vi "Text_New.vi"(7 "CreateMethod(Create or look up existing)":T1(ring), 8 "error in (no error)":errorcluster, 10 "Object name":string, 11 "Text In":refnum<class "Text.lvclass">) -> (0 "error out":errorcluster, 2 "DVRRefOut":refnum<data-value>, 3 "Text Out":refnum<class "Text.lvclass">, 5 "NewObjectCreated":bool)   [LabVIEW 2015, in "Front Panel Publisher.lvlib" / "Text.lvclass"]
uses:
  Text.lvclass
  Attributes.ctl
  Text.lvclass/Text.ctl
  Object_class/Object.lvclass
panel:
  in  "DVRRef(Hidden)":refnum<data-value>
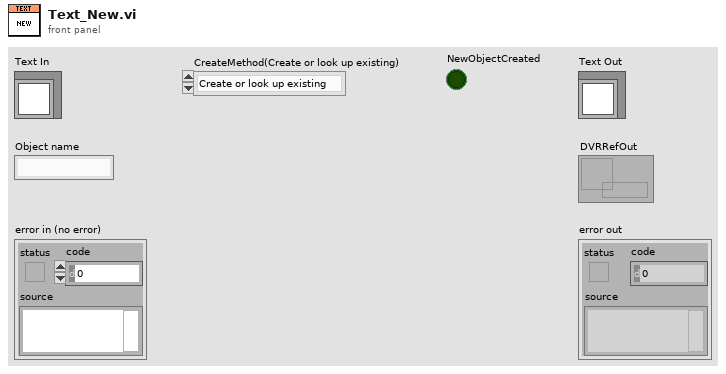
[diagram p1: front panel]
types:
  T1 = enum16{"Create or look up existing", "Look up existing"}
  T2 = typedef "Front Panel Publisher.lvlib/Text.lvclass/Attributes.ctl" = cluster{"Text":string, "Font":string, "Font Size":u32, "Visible":bool, "Control Reference":refnum<vi>}
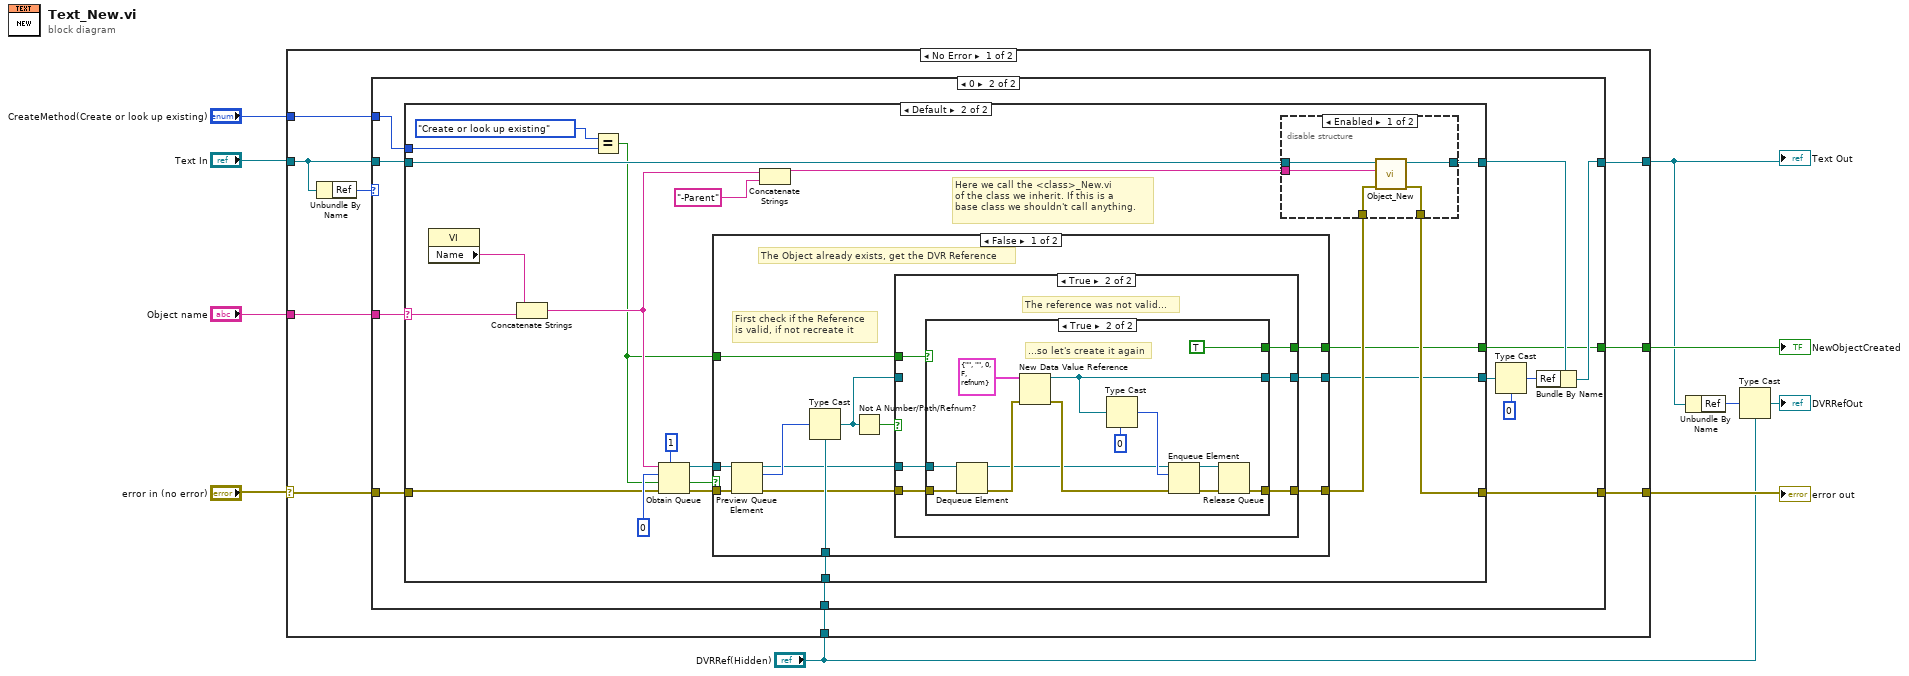
[diagram p0: block diagram]
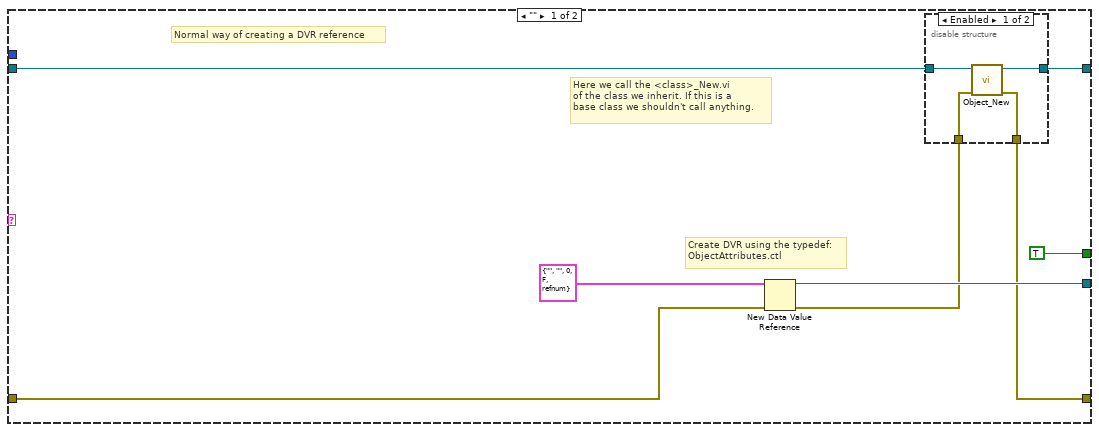
[diagram p3: hidden frame]
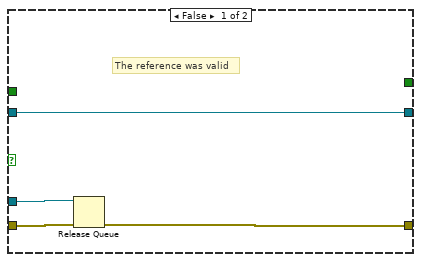
[diagram p5: hidden frame]
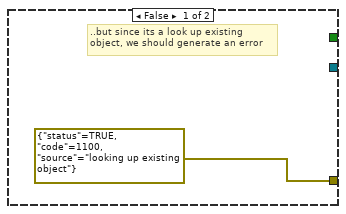
[diagram p6: hidden frame]
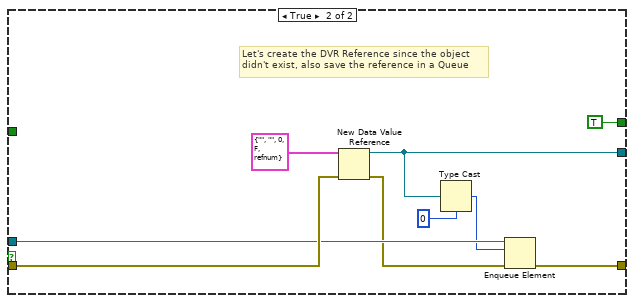
[diagram p7: hidden frame]
diagram:
  n1 = case shown="No Error" "error in (no error)" {
    selector: "error in (no error)" -> [w19 w122]
    tunnel: [w16 w122] -> w6
    tunnel: "CreateMethod(Create or look up existing)" -> [w17 _]
    tunnel: "Object name" -> [w18 _]
    tunnel: "DVRRef(Hidden)" -> [w15 _]
    tunnel: "Text In" -> [w14 w121]
    tunnel: [w13 w121] -> w3
    tunnel: [w12 _] -> w5
    frame No Error {
      n2 = Unbundle By Name(w14) -> ("Ref"=w11:u32)
      n3 = case shown="0" w11 {
        tunnel: w19 -> [w21 w33]
        tunnel: w18 -> [_ w32]
        tunnel: w17 -> [_ w31]
        tunnel: [w21 w30] -> w16
        tunnel: w14 -> [w20 w28]
        tunnel: [w20 w29] -> w13
        tunnel: w15 -> [_ w26]
        tunnel: [_ w25] -> w12
        frame Default {
          # "The DVR reference has already been created, from this child class's <Child>_New.vi"
        }
        frame 0 {
          n4 = case shown="Default" w32 {
            selector: w32 -> [_ w60]
            tunnel: w33 -> [w41 w57]
            tunnel: [w36 w58] -> w30
            tunnel: w31 -> [_ w67]
            tunnel: [w40 w51] -> w23
            tunnel: w28 -> [w39 w66]
            tunnel: [w38 w65] -> w27
            tunnel: w26 -> [_ w56]
            tunnel: [TRUE w50] -> w25
            frame "" {
              # "Create DVR using the typedef:\nObjectAttributes.ctl"
              # "Here we call the <class>_New.vi\nof the class we inherit. If this is a\nbase class we shouldn't call anything."
              # "Normal way of creating a DVR reference"
              n5 = New Data Value Reference(data value=T2 {"Text"="", "Font"="", "Font Size"=0, "Visible"=FALSE, "Control Reference"=refnum} ("Data"), error in=w41) -> (data value reference=w40:refnum<data-value>, error out=w37:errorcluster)
              n6 = disable-structure shown="Enabled" {
                disable-tunnel: w39 -> [w45 w47]
                disable-tunnel: [w44 w47] -> w38
                disable-tunnel: w37 -> [w43 w46]
                disable-tunnel: [w42 w46] -> w36
                frame Enabled {
                  n7 = call "Object_New.vi"("error in (no error)"=w43, "Object In"=w45) -> ("error out"=w42:errorcluster, "Object Out"=w44:refnum<class "Text.lvclass">)  [unwired: 6 in, 2 out]
                }
                frame Disabled {
                }
              }
            }
            frame Default {
              # "Here we call the <class>_New.vi\nof the class we inherit. If this is a\nbase class we shouldn't call anything."
              n8 = property class="VI"() -> ("Name"=w61:string)  [unwired: 2 in, 2 out]
              n9 = Concatenate Strings(w61, w60) -> (w59:string)
              n10 = Equal?(x=T1."Create or look up existing", y=w67) -> (x = y?=w49:bool)
              n11 = Obtain Queue(max queue size (-1, unlimited)=1, name (unnamed)=w59, element data type=u32 0 ("DataRef"), create if not found? (T)=w49, error in (no error)=w57) -> (queue out=w54:refnum<queue>, created new?=w53:bool, error out=w55:errorcluster)
              n12 = case shown="False" w53 {
                tunnel: w55 -> [w79 w113]
                tunnel: w54 -> [w80 w112]
                tunnel: [w74 w109] -> w52
                tunnel: [w72 w108] -> w51
                tunnel: w56 -> [w77 _]
                tunnel: [w70 TRUE] -> w50
                tunnel: w49 -> [w69 _]
                frame False {
                  # "First check if the Reference\nis valid, if not recreate it"
                  # "The Object already exists, get the DVR Reference"
                  n13 = Preview Queue Element(queue=w80, error in (no error)=w79) -> (queue out=w71:refnum<queue>, element=w78:u32, error out=w76:errorcluster)  [unwired: 1 in, 1 out]
                  n14 = Type Cast(type=w77, x=w78) -> (*(type *) &x=w73:refnum<data-value>)
                  n15 = Not A Number/Path/Refnum?(number/path/refnum=w73) -> (NaN/Path/Refnum?=w75:bool)
                  n16 = case shown="True" w75 {
                    tunnel: w76 -> [w82 w89]
                    tunnel: [w81 w87] -> w74
                    tunnel: w73 -> [w84 _]
                    tunnel: [w84 w88] -> w72
                    tunnel: w71 -> [w83 w90]
                    tunnel: [_ w86] -> w70
                    tunnel: w69 -> [_ w85]
                    frame False {
                      # "The reference was valid"
                      n17 = Release Queue(queue=w83, error in (no error)=w82) -> (error out=w81:errorcluster)  [unwired: 1 in, 2 out]
                    }
                    frame True {
                      # "The reference was not valid..."
                      n18 = case shown="True" w85 {
                        tunnel: w90 -> [_ w104]
                        tunnel: w89 -> [_ w103]
                        tunnel: [_ w97] -> w88
                        tunnel: [errorcluster {"status"=TRUE, "code"=1100, "source"="looking up existing object"} ("error out") w93] -> w87
                        tunnel: [_ TRUE] -> w86
                        frame False {
                          # "..but since its a look up existing\nobject, we should generate an error"
                        }
                        frame True {
                          # "...so let's create it again"
                          n19 = Dequeue Element(queue=w104, error in (no error)=w103) -> (queue out=w98:refnum<queue>, error out=w100:errorcluster)  [unwired: 1 in, 2 out]
                          n20 = New Data Value Reference(data value=T2 {"Text"="", "Font"="", "Font Size"=0, "Visible"=FALSE, "Control Reference"=refnum} ("Data"), error in=w100) -> (data value reference=w97:refnum<data-value>, error out=w99:errorcluster)
                          n21 = Type Cast(type=u32 0 ("ObjectQueue"), x=w97) -> (*(type *) &x=w101:u32)
                          n22 = Enqueue Element(queue=w98, element=w101, error in (no error)=w99) -> (queue out=w95:refnum<queue>, error out=w94:errorcluster)  [unwired: 1 in, 1 out]
                          n23 = Release Queue(queue=w95, error in (no error)=w94) -> (error out=w93:errorcluster)  [unwired: 1 in, 2 out]
                        }
                      }
                    }
                  }
                }
                frame True {
                  # "Let's create the DVR Reference since the object\ndidn't exist, also save the reference in a Queue"
                  n24 = New Data Value Reference(data value=T2 {"Text"="", "Font"="", "Font Size"=0, "Visible"=FALSE, "Control Reference"=refnum} ("Data"), error in=w113) -> (data value reference=w108:refnum<data-value>, error out=w110:errorcluster)
                  n25 = Type Cast(type=u32 0 ("ObjectQueue"), x=w108) -> (*(type *) &x=w107:u32)
                  n26 = Enqueue Element(queue=w112, element=w107, error in (no error)=w110) -> (error out=w109:errorcluster)  [unwired: 1 in, 2 out]
                }
              }
              n27 = Concatenate Strings(w59, "-Parent" ("string")) -> (w62:string)
              n28 = disable-structure shown="Enabled" {
                disable-tunnel: w66 -> [w118 w120]
                disable-tunnel: [w117 w120] -> w65
                disable-tunnel: w62 -> [w116 _]
                disable-tunnel: w52 -> [w115 w119]
                disable-tunnel: [w114 w119] -> w58
                frame Enabled {
                  n29 = call "Object_New.vi"("error in (no error)"=w115, "Object name"=w116, "Object In"=w118) -> ("error out"=w114:errorcluster, "Object Out"=w117:refnum<class "Text.lvclass">)  [unwired: 5 in, 2 out]
                }
                frame Disabled {
                }
              }
            }
          }
          n30 = Type Cast(type=u32 0 ("DataRef"), x=w23) -> (*(type *) &x=w22:u32)
          n31 = Bundle By Name(cluster=w27, "Ref"=w22) -> (w29:refnum<class "Text.lvclass">)
        }
      }
    }
    frame Error {
    }
  }
  "error out" <- w6
  "Text Out" <- w3
  "NewObjectCreated" <- w5
  n32 = Unbundle By Name(w3) -> ("Ref"=w4:u32)
  n33 = Type Cast(type="DVRRef(Hidden)", x=w4) -> (*(type *) &x=→"DVRRefOut":refnum<data-value>)
